vi "主界面B010 - 副本.vi"() -> ()   [LabVIEW 2013]
uses:
  <vilib>/Utility/file.llb/Read From Spreadsheet File (string).vi
  PCI8622_32.dll
panel:
  in  "Y挡圈最大值":dbl
  in  "Y挡圈最小值":dbl
  in  "X挡圈最大值":dbl
  in  "X挡圈最小值":dbl
  in  "Y内圈最大值":dbl
  in  "Y内圈最小值":dbl
  in  "X内圈最大值":dbl
  in  "X内圈最小值":dbl
  in  "Y轴承最大值":dbl
  in  "Y轴承最小值":dbl format="%#_13g"
  in  "X轴承最大值":dbl=12.0 format="%#_13g"
  in  "X轴承最小值":dbl=1.0 format="%#_13g"
  out "数值":i32
  out "员工ID":string
  out "压铆最大压力(N)":dbl
  out "压铆最小压力(N)":dbl
  out "3最大压装位移":dbl
  out "3最小压装位移":dbl
  out "3监控点":dbl
  in  "压轴承换向压力":dbl=5000.0
  out "换向指示1":bool
  in  "报警工步号":dbl
  out "报警提示":string
  in  "轴承压头速度（手动）":dbl
  in  "轴承压头位置（手动）":dbl
  in  "轴承内圈压头速度（手动）":dbl
  in  "轴承内圈压头位置（手动）":dbl
  out "换向指示2":bool
  in  "换向压力2":dbl=5000.0
  in  "工步号复位":bool
  out "通讯状态":bool
  in  "电动缸2ARST":bool
  in  "电动缸1ARST":bool
  out "内圈压头位置(mm)":dbl format="%#.1f"
  out "轴承压头位置(mm)":dbl format="%#.1f"
  out "型号数量":i32
  out "轴承压头位移(mm)":dbl format="%#.1f"
  out "内圈位移(mm)":dbl format="%#.1f"
  out "压铆位移(mm)":dbl format="%#.1f"
  out "压铆压力(N)":dbl format="%#.1f"
  out "error out 4":errorcluster
  out "error out 3":errorcluster
  out "error out 2":errorcluster
  out "ADODB._Connection Out":refnum<k7>
  out "error out":errorcluster
  out "B010本序不合格":bool
  out "内圈压力(N)":dbl format="%#.1f"
  out "轴承压头压力(N)":dbl format="%#.1f"
  out "B010本序合格":bool
  in  "停止":bool
  in  "自动工步号":dbl
  out "产品选型":dbl
  out "芯片ID":string
  out "自动操作状态":string
  in  "联线按钮":bool
  in  "选项卡控件":T1(tab)
  out "轴承区域最小压力(N)":dbl
  out "轴承区域最大压力(N)":dbl
  out "压轴承最大压力(N)":dbl
  out "轴承压装位移(mm)":dbl
  out "轴承最小压装位移(mm)":dbl
  out "轴承最大压装位移(mm)":dbl
  out "轴承监控点":dbl
  out "压装轴承，挡圈曲线":cluster{"Y":dbl[], "Y":dbl[]}[](graph) caption="压球涨堵头1"
  out "轴承最小压力(N)":dbl
  out "轴承最大压力(N)":dbl
  out "压装轴承合格":bool
  out "压装轴承不合格":bool
  out "轴承监控点压力(N)":dbl
  out "内圈区域压力最大值(N)":dbl
  out "内圈区域压力最小值(N)":dbl
  out "内圈压装最大压力(N)":dbl
  out "压装滚针轴承":cluster{"Y":dbl[], "Y":dbl[]}[](graph) caption="压球涨堵头1"
  out "压内圈不合格":bool
  out "压内圈合格":bool
  out "内圈最大压力(N)":dbl
  out "内圈最小压力(N)":dbl
  out "内圈监控点":dbl
  out "内圈最大压装位移(mm)":dbl
  out "内圈最小压装位移(mm)":dbl
  out "内圈实测压装位移(mm)":dbl
  out "内圈监控点压力(N)":dbl
  out "压铆区域内最大压力(N)":dbl
  out "压铆区域内最小压力(N)":dbl
  out "挡圈压铆":cluster{"Y":dbl[], "Y":dbl[]}[](graph) caption="压球涨堵头1"
  out "压挡圈合格":bool
  out "压挡圈不合格":bool
  out "压铆最大压力(N)":dbl
  out "压铆压装位移(mm)":dbl
  out "轴承正面":bool
  in  "伺服2P 启动":bool
  in  "伺服1P 启动":bool
  in  "快速上升速度":dbl
  in  "快速上升位置":dbl
  in  "慢速下降速度":dbl
  in  "慢速下降位置":dbl
  in  "快速下降速度":dbl
  in  "快速下降位置":dbl
  in  "快速上升速度":dbl
  in  "快速上升位置":dbl
  in  "慢速下降速度":dbl
  in  "慢速下降位置":dbl
  in  "快速下降速度":dbl
  in  "伺服2回零":bool
  in  "伺服2上升":bool
  in  "伺服2下降":bool
  in  "伺服2复位":bool
  in  "快速下降位置":dbl
  in  "伺服1回零":bool
  in  "伺服1上升":bool
  in  "伺服1下降":bool
  in  "伺服1复位":bool
  out "急停按钮":bool
  out "联线状态":bool
  out "光幕保护":bool
  out "气压报警":bool
  out "滑台右位":bool
  out "滑台左位":bool
  in  "滑台右移":bool
  in  "滑台左移":bool
  in  "增压缸下压":bool
  in  "增压缸上升":bool
  in  "增压缸增压":bool
  in  "增压缸卸压":bool
  in  "压铆压力零点偏移":dbl format="%#.2f"
  in  "压铆压力比例偏移":dbl format="%#.2f"
  in  "压铆位移零点偏移":dbl format="%#.2f"
  in  "压铆位移比例偏移":dbl format="%#.2f"
  in  "内圈压力零点偏移":dbl format="%#.2f"
  in  "内圈压力比例偏移":dbl format="%#.2f"
  in  "内圈位移零点偏移":dbl format="%#.2f"
  in  "内圈位移比例偏移":dbl format="%#.2f"
  in  "轴承压力零点偏移":dbl format="%#.2f"
  in  "轴承压力比例偏移":dbl format="%#.2f"
  in  "轴承位移零点偏移":dbl format="%#.2f"
  in  "轴承位移比例偏移":dbl format="%#.2f"
  in  "传感器参数查询":bool
  in  "传感器参数保存":bool
  in  "参数浏览表":string[][](table)=[["J709", "J728", "J706"], ["1", "1", "1"], ["168", "78.5", "98"], ["0", "500", "500"], ["10000", "5000", "5000"], ["0", "78", "97"], ["173", "80", "102"], ["183", "85.5", "79"], ["0", "500", "500"], ["20000", "5000", "5000"], ["0", "85.5", "83"], ["190", "86.5", "84"], ["250", "144", "144"], ["0", "55000", "55000"], ["100000", "65000", "65000"], ["0", "143", "143"], ["300", "147", "147"], ["-70", "-89\n", "-94"], ["20", "50", "50"], ["-80.95", "-104", "-113"], ["1", "1", "1"], ["0", "0", "0"], ["20", "50", "50"], ["-77", "-70", "-75"], ["20", "50", "50"], ["-92.5", "-82", "-87"], ["1", "1", "1"], ["0", "0", "0"], ["20", "50", "50"], ["1", "95", "97"], ["84", "96", "99"], ["2000", "500", "500"], ["4000", "5000", "5000"], ["81", "75", "79"], ["82", "77", "81"], ["0", "500", "500"], ["25000", "5000", "5000"], ["250", "184", "143"], ["252", "186", "144"], ["10000", "10000", "10000"], ["60000", "50000", "50000"], ["", "5000", "5000"], ["", "5000", "5000"], ["", "93", "93"], ["", "100", "102"], ["", "-10", "-10"], ["", "10000", "10000"], ["", "71", "77"], ["", "80", "85"], ["", "-10", "-10"], ["", "6000", "6000"], ["", "180", ""], ["", "190", ""], ["", "-10", ""], ["", "70000", ""]]
  in  "参数查询":bool
  in  "试验参数保存":bool
  in  "轴承区域最小位移(mm)":dbl=84.0
  in  "轴承区域最大位移(mm)":dbl=85.0
  in  "轴承区域最小压力(N)":dbl=500.0
  in  "轴承区域最大压力(N)":dbl=5000.0
  in  "内圈区域最小位移(mm)":dbl=90.0
  in  "内圈区域最大位移(mm)":dbl=91.0
  in  "内圈区域最小压力(N)":dbl=500.0
  in  "内圈区域最大压力(N)":dbl=5000.0
  in  "挡圈区域最小位移(mm)":dbl=250.0
  in  "挡圈区域最大位移(mm)":dbl=252.0
  in  "挡圈区域最小压力(N)":dbl=10000.0
  in  "挡圈区域最大压力(N)":dbl=60000.0
  out "员工姓名":string
  in  "型号选择":u16(ring)=1 items=["J709", "J728", "J706"]
  in  "参数加载":bool
  out "产品ID":string
  # "判定参数"
  # "芜湖机械转向器装配线"
  # "齿轮轴总成装配"
  # "Q14070机械转向器装配线"
  # "湖北唯思凌科装备制造有限公司 设计开发 (C)2015"
  # "判定参数"
  # "实测值"
  # "判定参数"
  # "实测值"
  # "实测值"
  # "轴承\n压头\n设置"
  # "轴承\n内圈\n压头\n设置"
  # "传感器校验区"
  # "注意：\n具备权限的用户才能够修改传感器校验参数和试验参数！"
  # "关于传感器校验：\n1、传感器校验需要由具备资质的单位或部门进行校验。\n2、具备权限的用户才能够修改传感器校验参数和试验参数。\n3、修改校验参数方法：先将比例偏移置为1，修改零点偏移，使零点值与校验的传感器一致；然后根据增幅调整比例偏移。"
  # "注意：\n具备权限的用户才能够修改传感器校验参数和试验参数！"
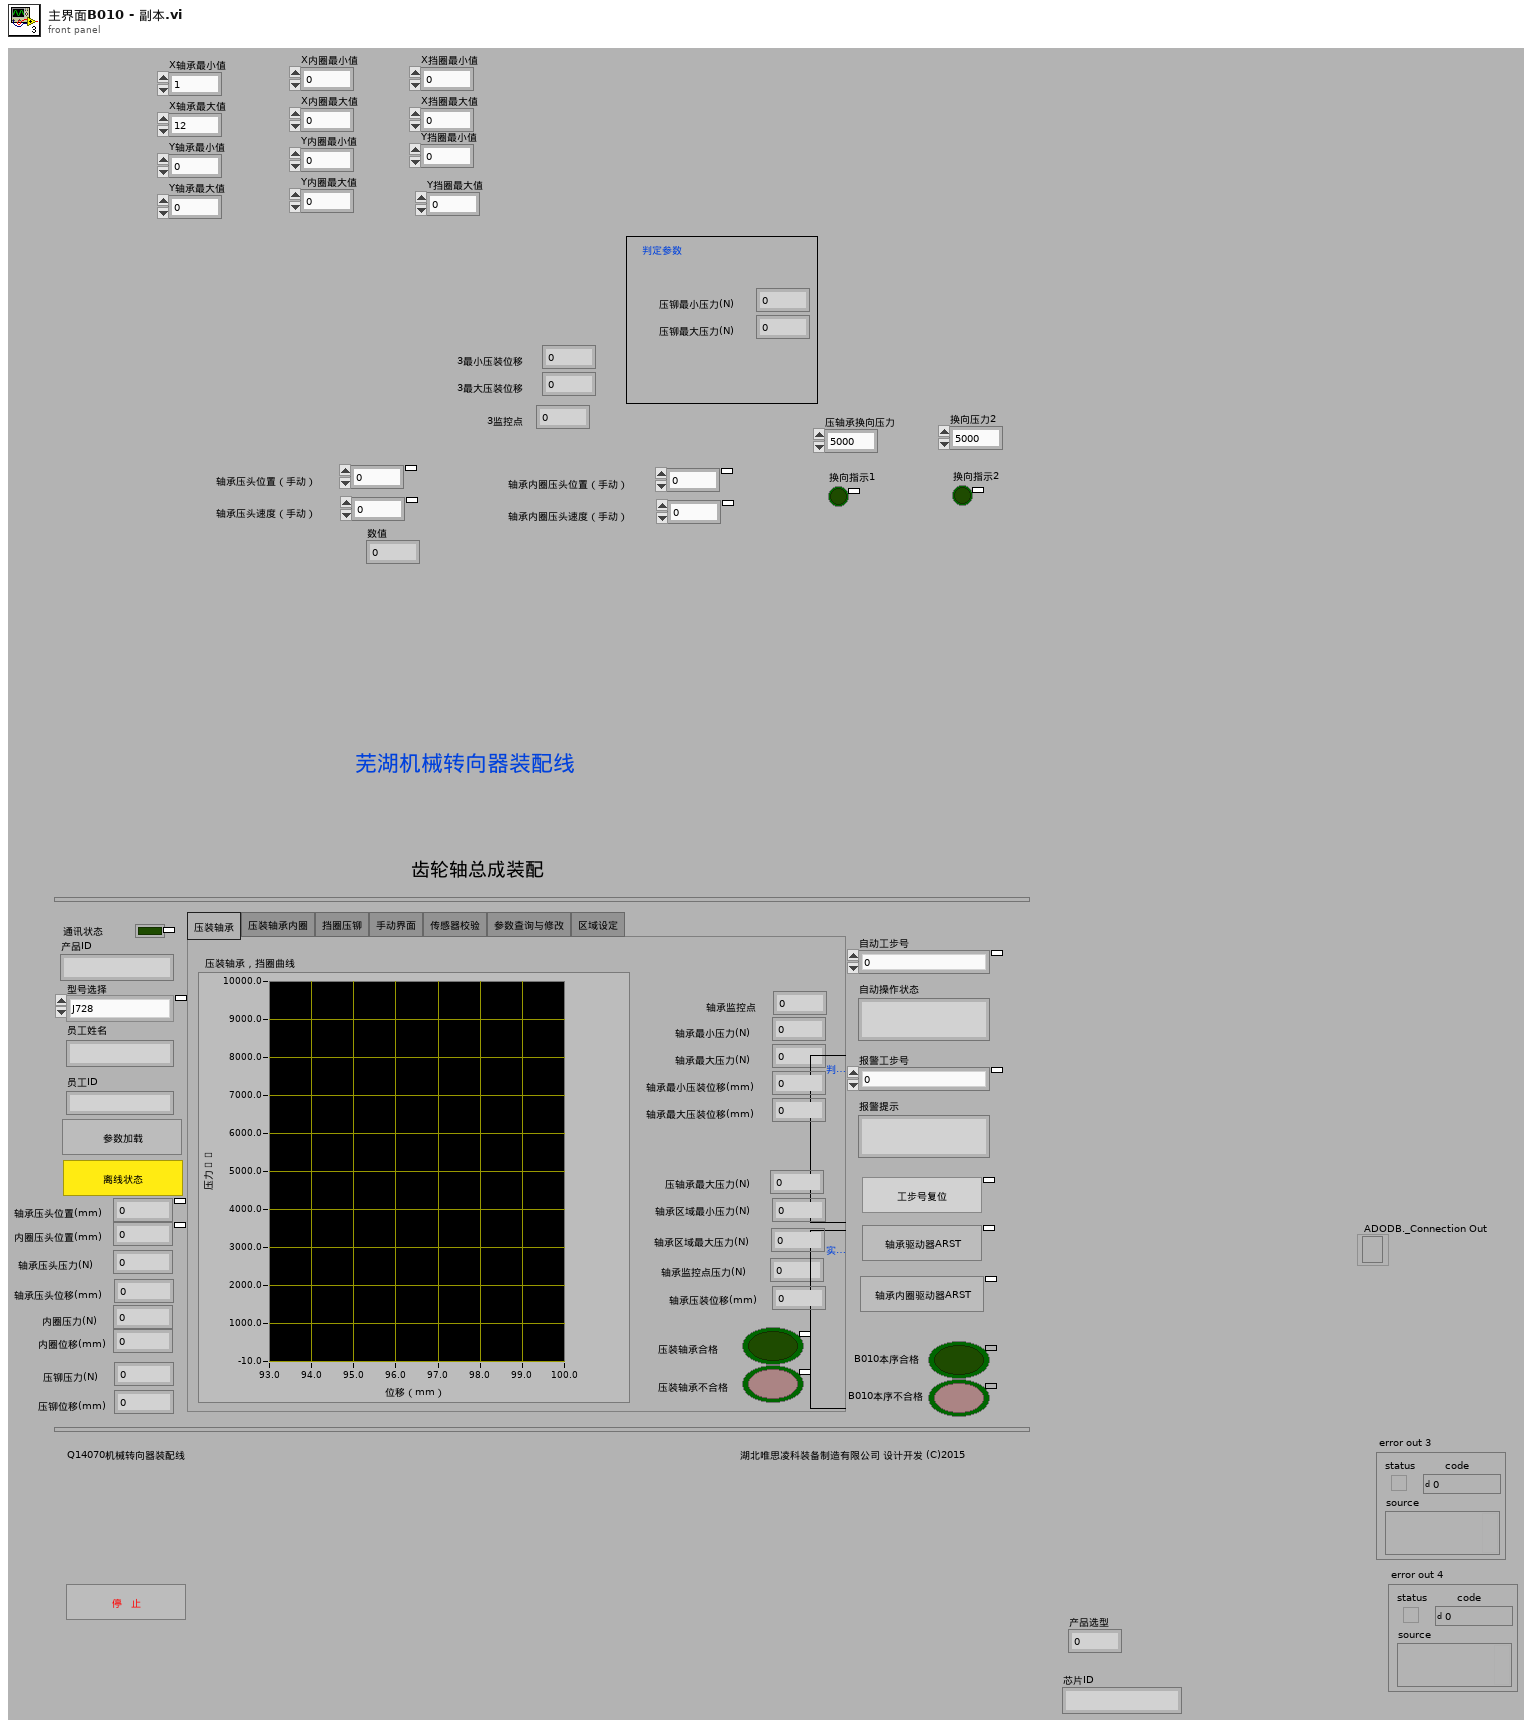
[diagram p1: front panel]
types:
  T1 = enum32{"压装轴承", "压装轴承内圈", "挡圈压铆", "手动界面", "传感器校验", "参数查询与修改", "区域设定"}
  T2 = typedef "imagedata.ctl" = cluster{"image type":i32, "image depth":i32, "image":u8[], "mask":u8[], "colors":u32[], "Rectangle":cluster{"left":i16, "top":i16, "right":i16, "bottom":i16}}
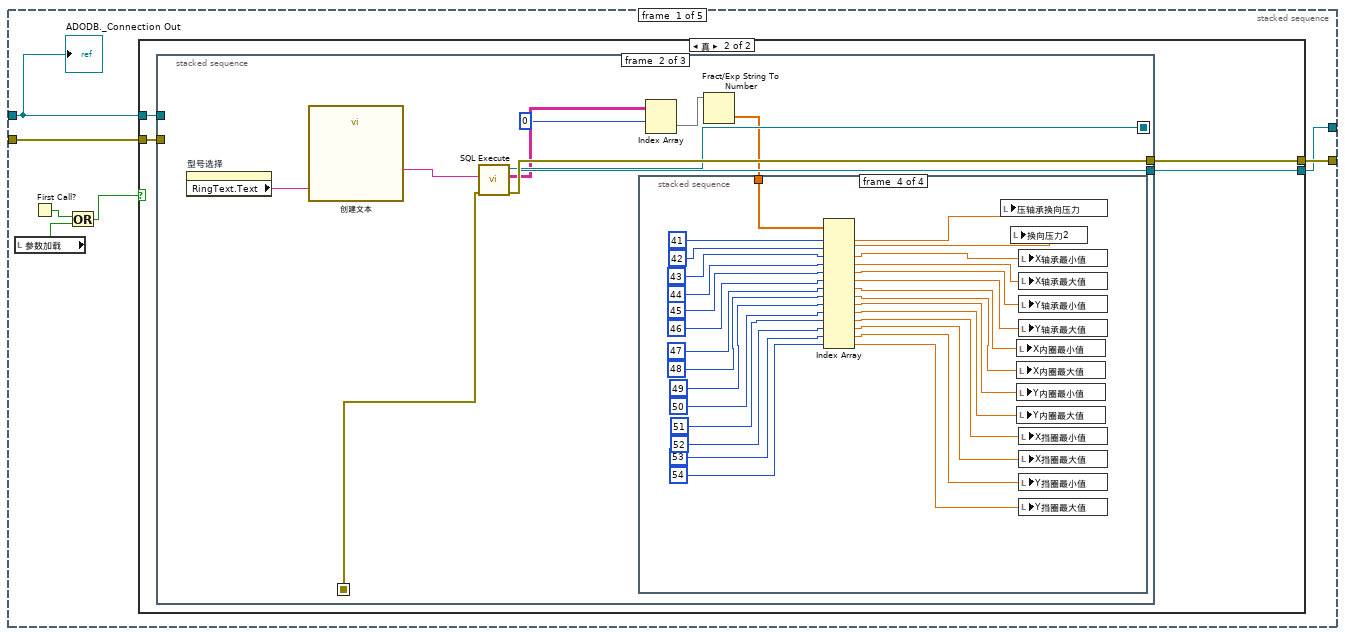
[diagram p2: hidden frame]
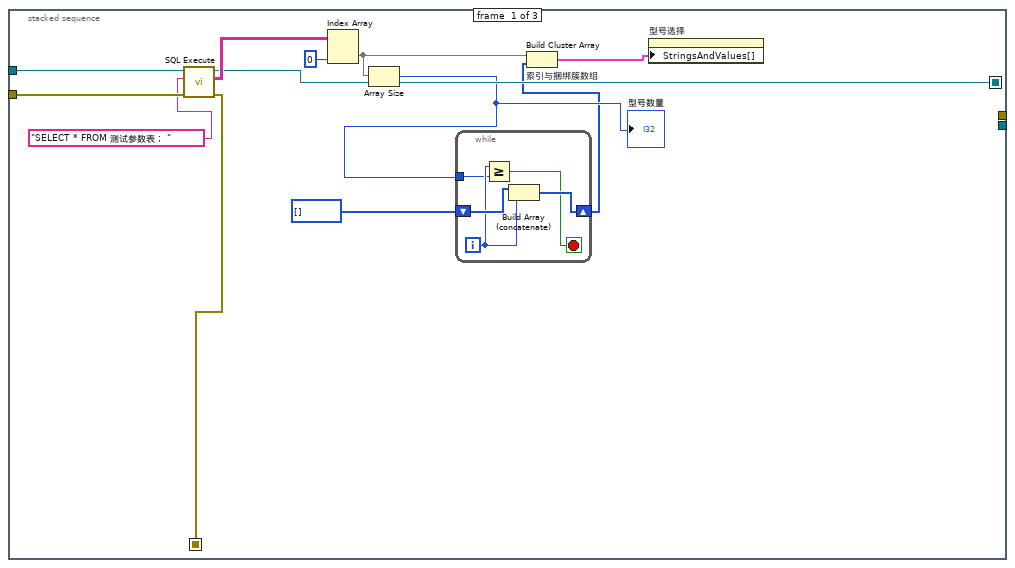
[diagram p4: hidden frame]
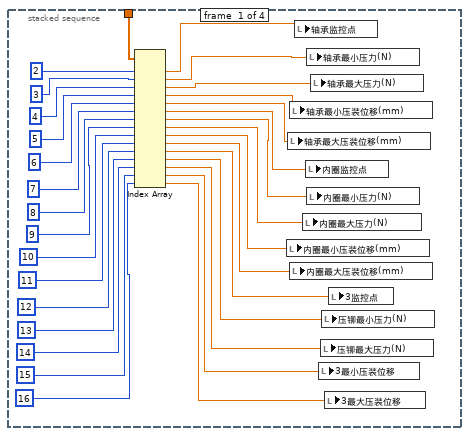
[diagram p5: hidden frame]
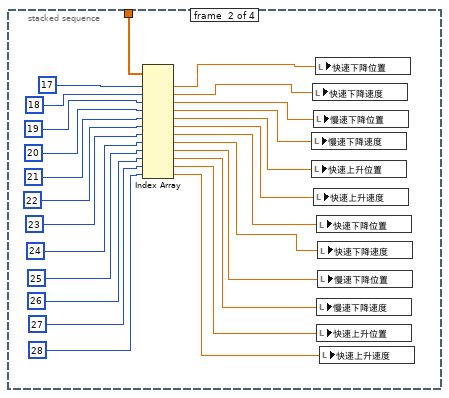
[diagram p6: hidden frame]
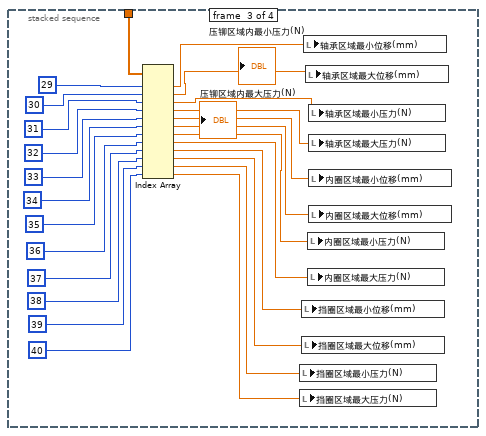
[diagram p7: hidden frame]
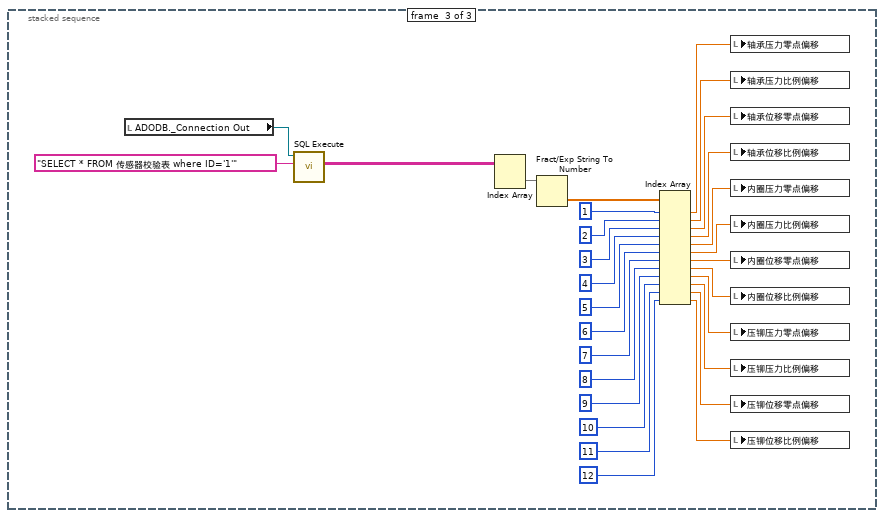
[diagram p8: hidden frame]
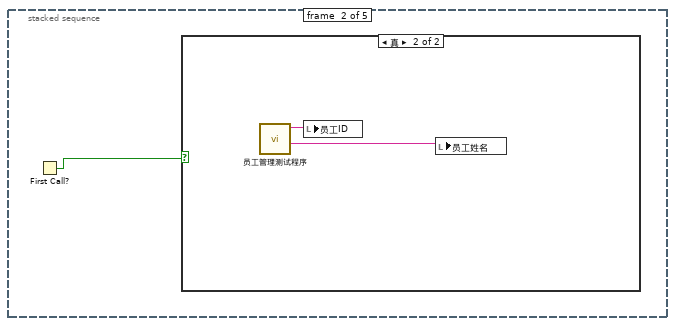
[diagram p9: hidden frame]
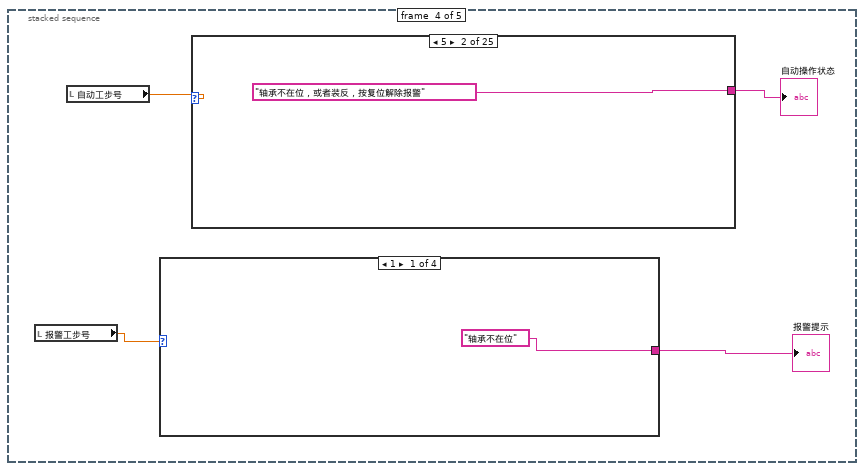
[diagram p11: hidden frame]
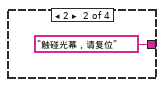
[diagram p12: hidden frame]
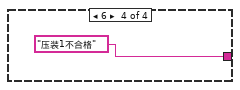
[diagram p14: hidden frame]
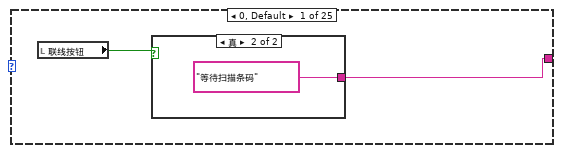
[diagram p15: hidden frame]
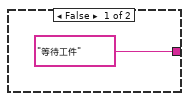
[diagram p16: hidden frame]
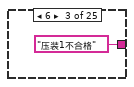
[diagram p17: hidden frame]
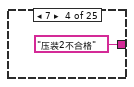
[diagram p18: hidden frame]
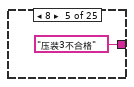
[diagram p19: hidden frame]
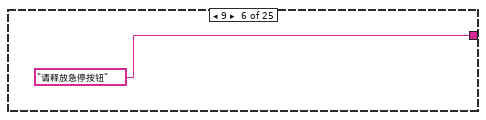
[diagram p20: hidden frame]
diagram:
  n1 = while {
    stop <- w10 stop-if-true
    n2 = local read "自动工步号"() -> (w8:dbl)
    n3 = Wait Until Next ms Multiple(millisecond multiple=u32 100 ("毫秒倍数")) -> ()  [unwired: 1 out]
    n4 = case shown="60" w8 {
      frame 0, Default {
      }
      frame 10 {
        n5 = flat-sequence {
          tunnel: [w25] -> w16
          tunnel: [w33] -> w22
          tunnel: [w32] -> w21
          tunnel: w16 -> [w31]
          tunnel: w22 -> [w59]
          tunnel: w21 -> [w57]
          tunnel: [w65] -> w20
          tunnel: [w64] -> w19
          tunnel: [w58] -> w14
          tunnel: w20 -> [w73]
          tunnel: w19 -> [w78]
          tunnel: [w75] -> w18
          tunnel: [w71] -> w17
          tunnel: [w70] -> w15
          tunnel: w14 -> [w70]
          tunnel: [w69] -> w13
          tunnel: [w68] -> w12
          tunnel: w18 -> [w87]
          tunnel: w17 -> [w86]
          tunnel: w15 -> [w83]
          tunnel: w13 -> [w85]
          tunnel: w12 -> [w84]
          tunnel: [w79] -> w11
          tunnel: w11 -> [w89]
          frame #0 {
            w23 = FALSE ("换向指示1")
            w30 = FALSE
            n6 = local write "压装轴承不合格"(w30) -> ()
            n7 = local write "压装轴承合格"(w30) -> ()
            n8 = property on="轴承监控点压力(N)" class="DigNum (严格)"("Blinking"=w23) -> ()  [unwired: 2 in, 2 out]
            n9 = local write "换向指示1"(w23) -> ()
            n10 = local write "换向指示2"(w23) -> ()
            n11 = local write "选项卡控件"(T1."压装轴承" ("选项卡控件")) -> ()
            n12 = call "区域曲线.vi"("区域最大压力(N)"="轴承区域最大压力(N)", "区域最小压力(N)"="轴承区域最小压力(N)", "区域最大位移(mm)"="轴承区域最大位移(mm)", "区域最小位移(mm)"="轴承区域最小位移(mm)") -> ("区域曲线"=w25:cluster{dbl[], dbl[]})  [unwired: 7 in]
          }
          frame #1 {
            w34 = dbl[] []
            n13 = while {
              shift-right: [w52] -> w33
              shift-left: w34 -> [w53]
              shift-right: [w50] -> w32
              shift-left: w34 -> [w51]
              tunnel: w31 -> [w40]
              stop <- w36 stop-if-true
              n14 = local read "轴承压头位置(mm)"() -> (w43:dbl)
              n15 = local read "自动工步号"() -> (w46:dbl)
              n16 = local read "轴承压头压力(N)"() -> (w49:dbl)
              n17 = local read "轴承压头压力(N)"() -> (w39:dbl)
              n18 = local read "压轴承换向压力"() -> (w38:dbl)
              n19 = Equal?(x=w46, y=30.0) -> (x = y?=w37:bool)
              n20 = Multiply(x=w43, y=-1.0) -> (x*y=w41:dbl)
              n21 = Build Array (concatenate)(w53, w41) -> (w52:dbl[])
              n22 = Build Array (concatenate)(w51, w49) -> (w50:dbl[])
              n23 = Bundle(w52, w50) -> (w48:cluster{dbl[], dbl[]})  [unwired: 1 in]
              n24 = Greater Or Equal?(x=w39, y=w38) -> (x >= y?=w35:bool)
              n25 = Build Array(w48, w40) -> (w47:cluster{dbl[], dbl[]}[])
              n26 = Or(x=w37, y=w35) -> (x .or. y?=w36:bool)
              n27 = local write "压装轴承，挡圈曲线"(w47) -> ()
              n28 = Wait Until Next ms Multiple(millisecond multiple=u32 50 ("毫秒倍数")) -> ()  [unwired: 1 out]
              n29 = local write "换向指示1"(w35) -> ()
            }
          }
          frame #2 {
            n30 = local read "轴承监控点"() -> (w67:dbl)
            n31 = local read "轴承区域最大位移(mm)"() -> (w62:dbl)
            n32 = local read "轴承区域最小位移(mm)"() -> (w63:dbl)
            n33 = local read "轴承区域最小压力(N)"() -> (w61:dbl)
            n34 = local read "轴承区域最大压力(N)"() -> (w60:dbl)
            n35 = Array Max & Min(array=w59) -> (max value=w64:dbl)  [unwired: 3 out]
            n36 = Array Max & Min(array=w57) -> (max value=→"压轴承最大压力(N)":dbl)  [unwired: 3 out]
            n37 = Threshold 1D Array "以阈值插值一维数组"(2:w67, 3:w59) -> (0:w66:dbl)  [unwired: 1 in]
            n38 = local write "轴承压装位移(mm)"(w64) -> ()
            n39 = Index Array(array=w57, index=w66) -> (element=w65:dbl)
            n40 = call "区域判断.vi"("压力数组"=w57, "位移数组"=w59, "区域最大压力"=w60, "区域最小压力"=w61, "区域最大位移"=w62, "区域最小位移"=w63) -> ("数值 2"=→"轴承区域最小压力(N)":dbl, "数值"=→"轴承区域最大压力(N)":dbl, "区域监控合格"=w58:bool)  [unwired: 1 in]
            n41 = local write "轴承监控点压力(N)"(w65) -> ()
          }
          frame #3 {
            n42 = local read "轴承最大压装位移(mm)"() -> (w77:dbl)
            n43 = local read "轴承最小压装位移(mm)"() -> (w76:dbl)
            n44 = local read "轴承最大压力(N)"() -> (w72:dbl)
            n45 = local read "轴承最小压力(N)"() -> (w74:dbl)
            n46 = In Range and Coerce(upper limit=w77, x=w78, lower limit=w76) -> (In Range?=w69:bool)  [unwired: 1 out]
            n47 = In Range and Coerce(upper limit=w72, x=w73, lower limit=w74) -> (In Range?=w68:bool)  [unwired: 1 out]
            n48 = Not(x=w69) -> (.not. x?=w75:bool)
            n49 = Not(x=w68) -> (.not. x?=w71:bool)
          }
          frame #4 {
            n50 = property on="轴承监控点压力(N)" class="DigNum (严格)"("Blinking"=w86) -> ()  [unwired: 2 in, 2 out]
            n51 = property on="轴承压装位移(mm)" class="DigNum (严格)"("Blinking"=w87) -> ()  [unwired: 2 in, 2 out]
            n52 = Compound Arithmetic op=AND(w85, w84, w83) -> (w82:bool)
            "压装轴承合格" <- w82
            n53 = Not(x=w82) -> (.not. x?=w81:bool)
            "压装轴承不合格" <- w81
            n54 = Wait Until Next ms Multiple(millisecond multiple=u32 80 ("毫秒倍数")) -> ()  [unwired: 1 out]
            n55 = local read "联线按钮"() -> (w80:bool)
            n56 = And(x=w81, y=w80) -> (x .and. y?=w79:bool)
          }
          frame #5 {
            n57 = case shown="真" w89 {
              frame False {
              }
              frame True {
                n58 = local write "B010本序不合格"(TRUE ("B010本序不合格")) -> ()
                n59 = local write "B010本序合格"(FALSE ("B010本序合格")) -> ()
              }
            }
          }
        }
      }
      frame 60 {
        n60 = flat-sequence {
          tunnel: [w107] -> w98
          tunnel: [w114] -> w104
          tunnel: [w113] -> w103
          tunnel: w98 -> [w112]
          tunnel: w104 -> [w140]
          tunnel: w103 -> [w138]
          tunnel: [w146] -> w102
          tunnel: [w145] -> w101
          tunnel: [w139] -> w96
          tunnel: w102 -> [w157]
          tunnel: w101 -> [w159]
          tunnel: [w158] -> w100
          tunnel: [w156] -> w99
          tunnel: [w151] -> w97
          tunnel: w96 -> [w151]
          tunnel: [w150] -> w95
          tunnel: [w149] -> w94
          tunnel: w100 -> [w167]
          tunnel: w99 -> [w166]
          tunnel: w97 -> [w165]
          tunnel: w95 -> [w164]
          tunnel: w94 -> [w163]
          tunnel: [w161] -> w93
          tunnel: [w160] -> w92
          tunnel: w93 -> [w171]
          tunnel: w92 -> [w170]
          frame #0 {
            w105 = FALSE
            n61 = property on="内圈监控点压力(N)" class="DigNum (严格)"("Blinking"=w105) -> ()  [unwired: 2 in, 2 out]
            n62 = local write "压内圈合格"(w105) -> ()
            n63 = local write "压内圈不合格"(w105) -> ()
            n64 = local write "换向指示2"(w105) -> ()
            n65 = local write "选项卡控件"(T1."压装轴承内圈" ("选项卡控件")) -> ()
            n66 = call "区域曲线.vi"("区域最大压力(N)"="内圈区域最大压力(N)", "区域最小压力(N)"="内圈区域最小压力(N)", "区域最大位移(mm)"="内圈区域最大位移(mm)", "区域最小位移(mm)"="内圈区域最小位移(mm)") -> ("区域曲线"=w107:cluster{dbl[], dbl[]})  [unwired: 7 in]
          }
          frame #1 {
            w115 = dbl[] []
            n67 = while {
              shift-right: [w133] -> w114
              shift-left: w115 -> [w134]
              shift-right: [w131] -> w113
              shift-left: w115 -> [w132]
              tunnel: w112 -> [w120]
              stop <- w119 stop-if-true
              n68 = local read "内圈压头位置(mm)"() -> (w122:dbl)
              n69 = local read "内圈压力(N)"() -> (w118:dbl)
              n70 = local read "内圈压力(N)"() -> (w121:dbl)
              n71 = local read "自动工步号"() -> (w129:dbl)
              n72 = Multiply(x=w122, y=-1.0) -> (x*y=w125:dbl)
              n73 = Build Array (concatenate)(w134, w125) -> (w133:dbl[])
              n74 = Build Array (concatenate)(w132, w121) -> (w131:dbl[])
              n75 = Equal?(x=w129, y=80.0) -> (x = y?=w127:bool)
              n76 = Greater Or Equal?(x=w118, y="换向压力2") -> (x >= y?=w116:bool)
              n77 = Or(x=w116, y=w127) -> (x .or. y?=w119:bool)
              n78 = Bundle(w133, w131) -> (w130:cluster{dbl[], dbl[]})  [unwired: 1 in]
              n79 = local write "换向指示2"(w116) -> ()
              n80 = Build Array(w130, w120) -> (w124:cluster{dbl[], dbl[]}[])
              n81 = local write "压装滚针轴承"(w124) -> ()
              n82 = Wait Until Next ms Multiple(millisecond multiple=u32 50 ("毫秒倍数")) -> ()  [unwired: 1 out]
            }
          }
          frame #2 {
            n83 = local read "内圈监控点"() -> (w147:dbl)
            n84 = local read "内圈区域最小位移(mm)"() -> (w144:dbl)
            n85 = local read "内圈区域最大位移(mm)"() -> (w143:dbl)
            n86 = local read "内圈区域最小压力(N)"() -> (w142:dbl)
            n87 = local read "内圈区域最大压力(N)"() -> (w141:dbl)
            n88 = Array Max & Min(array=w140) -> (max value=w145:dbl)  [unwired: 3 out]
            n89 = Array Max & Min(array=w138) -> (max value=→"内圈压装最大压力(N)":dbl)  [unwired: 3 out]
            n90 = Threshold 1D Array(2:w147, 3:w140) -> (0:w148:dbl)  [unwired: 1 in]
            n91 = Index Array(array=w138, index=w148) -> (element=w146:dbl)
            n92 = local write "内圈实测压装位移(mm)"(w145) -> ()
            n93 = local write "内圈监控点压力(N)"(w146) -> ()
            n94 = call "区域判断.vi"("压力数组"=w138, "位移数组"=w140, "区域最大压力"=w141, "区域最小压力"=w142, "区域最大位移"=w143, "区域最小位移"=w144) -> ("数值 2"=→"内圈区域压力最小值(N)":dbl, "数值"=→"内圈区域压力最大值(N)":dbl, "区域监控合格"=w139:bool)  [unwired: 1 in]
          }
          frame #3 {
            n95 = local read "内圈最大压装位移(mm)"() -> (w154:dbl)
            n96 = local read "内圈最小压装位移(mm)"() -> (w155:dbl)
            n97 = local read "内圈最大压力(N)"() -> (w153:dbl)
            n98 = local read "内圈最小压力(N)"() -> (w152:dbl)
            n99 = In Range and Coerce(upper limit=w154, x=w159, lower limit=w155) -> (In Range?=w150:bool)  [unwired: 1 out]
            n100 = In Range and Coerce(upper limit=w153, x=w157, lower limit=w152) -> (In Range?=w149:bool)  [unwired: 1 out]
            n101 = Not(x=w150) -> (.not. x?=w158:bool)
            n102 = Not(x=w149) -> (.not. x?=w156:bool)
          }
          frame #4 {
            n103 = property on="内圈监控点压力(N)" class="DigNum (严格)"("Blinking"=w166) -> ()  [unwired: 2 in, 2 out]
            n104 = property on="内圈实测压装位移(mm)" class="DigNum (严格)"("Blinking"=w167) -> ()  [unwired: 2 in, 2 out]
            n105 = Compound Arithmetic op=AND(w164, w165, w163) -> (w162:bool)
            n106 = Not(x=w162) -> (.not. x?=w161:bool)
            n107 = Wait Until Next ms Multiple(millisecond multiple=u32 80 ("毫秒倍数")) -> ()  [unwired: 1 out]
            n108 = local write "压内圈合格"(w162) -> ()
            n109 = local write "压内圈不合格"(w161) -> ()
            n110 = local read "联线按钮"() -> (w160:bool)
          }
          frame #5 {
            n111 = And(x=w171, y=w170) -> (x .and. y?=w169:bool)
            n112 = case shown="真" w169 {
              frame False {
              }
              frame True {
                n113 = local write "B010本序不合格"(TRUE ("B010本序不合格")) -> ()
                n114 = local write "B010本序合格"(FALSE ("B010本序合格")) -> ()
              }
            }
          }
        }
      }
      frame 110 {
        n115 = flat-sequence {
          tunnel: [w202] -> w190
          tunnel: [w194] -> w175
          tunnel: [w207] -> w193
          tunnel: [w206] -> w192
          tunnel: w190 -> [w205]
          tunnel: w175 -> [w204]
          tunnel: w193 -> [w227]
          tunnel: w192 -> [w228]
          tunnel: [w235] -> w183
          tunnel: [w236] -> w181
          tunnel: [w232] -> w179
          tunnel: [w231] -> w177
          tunnel: w183 -> [w242]
          tunnel: [w242] -> w182
          tunnel: w181 -> [w241]
          tunnel: [w241] -> w180
          tunnel: w179 -> [w240]
          tunnel: [w240] -> w178
          tunnel: w177 -> [w239]
          tunnel: [w239] -> w176
          tunnel: w182 -> [w255]
          tunnel: w180 -> [w257]
          tunnel: [w256] -> w191
          tunnel: w178 -> [w250]
          tunnel: [w250] -> w189
          tunnel: [w249] -> w188
          tunnel: [w248] -> w187
          tunnel: w176 -> [w245]
          tunnel: [w244] -> w184
          tunnel: [w243] -> w174
          tunnel: w191 -> [w266]
          tunnel: w189 -> [w260]
          tunnel: w188 -> [w261]
          tunnel: w187 -> [w265]
          tunnel: [w263] -> w186
          tunnel: [w262] -> w185
          tunnel: w184 -> [w259]
          tunnel: w174 -> [w258]
          tunnel: w186 -> [w270]
          tunnel: w185 -> [w269]
          frame #0 {
            w203 = FALSE
            n116 = local write "压挡圈不合格"(w203) -> ()
            n117 = local write "压挡圈合格"(w203) -> ()
            n118 = local write "选项卡控件"(T1."挡圈压铆" ("选项卡控件")) -> ()
            n119 = call "区域曲线.vi"("区域最大压力(N)"="挡圈区域最大压力(N)", "区域最小压力(N)"="挡圈区域最小压力(N)", "区域最大位移(mm)"="挡圈区域最大位移(mm)", "区域最小位移(mm)"="挡圈区域最小位移(mm)") -> ("区域曲线"=w202:cluster{dbl[], dbl[]})  [unwired: 7 in]
            n120 = call "区域曲线 - 副本.vi"("区域最大压力(N)"=100000.0, "区域最小压力(N)"=0.0, "区域最大位移(mm)"="挡圈区域最大位移(mm)", "区域最小位移(mm)"="挡圈区域最小位移(mm)") -> ("区域曲线1"=w194:cluster{dbl[], dbl[]})  [unwired: 7 in]
          }
          frame #1 {
            w208 = dbl[] []
            n121 = while {
              shift-right: [w211] -> w207
              shift-left: w208 -> [w223]
              shift-right: [w210] -> w206
              shift-left: w208 -> [w222]
              tunnel: w205 -> [w213]
              tunnel: w204 -> [w209]
              stop <- w218 stop-if-true
              n122 = local read "压铆压力(N)"() -> (w215:dbl)
              n123 = local read "压铆位移(mm)"() -> (w216:dbl)
              n124 = local read "自动工步号"() -> (w220:dbl)
              n125 = Build Array (concatenate)(w223, w216) -> (w211:dbl[])
              n126 = Build Array (concatenate)(w222, w215) -> (w210:dbl[])
              n127 = Equal?(x=w220, y=140.0) -> (x = y?=w218:bool)
              n128 = Bundle(w211, w210) -> (w221:cluster{dbl[], dbl[]})  [unwired: 1 in]
              n129 = Build Array(w221) -> (w214:cluster{dbl[], dbl[]}[])
              n130 = Build Array (concatenate)(w214, w213, w209) -> (w212:cluster{dbl[], dbl[]}[])
              n131 = Wait Until Next ms Multiple(millisecond multiple=u32 2 ("毫秒倍数")) -> ()  [unwired: 1 out]
              n132 = local write "挡圈压铆"(w212) -> ()
            }
          }
          frame #2 {
            n133 = local read "挡圈区域最小位移(mm)"() -> (w230:dbl)
            n134 = local read "挡圈区域最大位移(mm)"() -> (w229:dbl)
            n135 = local read "挡圈区域最大压力(N)"() -> (w233:dbl)
            n136 = local read "挡圈区域最小压力(N)"() -> (w234:dbl)
            n137 = local read "3监控点"() -> (w237:dbl)
            n138 = Array Max & Min(array=w227) -> (max value=w236:dbl)  [unwired: 3 out]
            n139 = Threshold 1D Array(2:w237, 3:w227) -> (0:w238:dbl)  [unwired: 1 in]
            n140 = Index Array(array=w228, index=w238) -> (element=w235:dbl)
            n141 = call "区域判断.vi"("压力数组"=w228, "位移数组"=w227, "区域最大压力"=w233, "区域最小压力"=w234, "区域最大位移"=w229, "区域最小位移"=w230) -> ("数值 2"=w226:dbl, "数值"=w225:dbl, "区域监控合格"=w232:bool)  [unwired: 1 in]
            n142 = local write "压铆压装位移(mm)"(w236) -> ()
            n143 = local write "压铆区域内最小压力(N)"(w226) -> ()
            n144 = local write "压铆区域内最大压力(N)"(w225) -> ()
            n145 = Array Max & Min(array=w228) -> (max value=w231:dbl)  [unwired: 3 out]
            n146 = local write "压铆最大压力(N)"(w231) -> ()
            n147 = property on="压铆最大压力(N)" class="DigNum (严格)"("Blinking"=FALSE ("闪烁")) -> ()  [unwired: 2 in, 2 out]
          }
          frame #3 {
          }
          frame #4 {
            n148 = local read "压铆最小压力(N)"() -> (w246:dbl)
            n149 = local read "挡圈区域最小压力(N)"() -> (w251:dbl)
            n150 = local read "压铆最大压力(N)"() -> (w247:dbl)
            n151 = local read "3最大压装位移"() -> (w254:dbl)
            n152 = local read "挡圈区域最大压力(N)"() -> (w252:dbl)
            n153 = local read "3最小压装位移"() -> (w253:dbl)
            n154 = In Range and Coerce(upper limit=w254, x=w257, lower limit=w253) -> (In Range?=w249:bool)  [unwired: 1 out]
            n155 = In Range and Coerce(upper limit=w252, x=w255, lower limit=w251) -> (In Range?=w248:bool)  [unwired: 1 out]
            n156 = In Range and Coerce(upper limit=w247, x=w245, lower limit=w246) -> (In Range?=w244:bool)  [unwired: 1 out]
            n157 = Not(x=w249) -> (.not. x?=w256:bool)
            n158 = Not(x=w244) -> (.not. x?=w243:bool)
          }
          frame #5 {
            n159 = property on="压铆最大压力(N)" class="DigNum (严格)"("Blinking"=w258) -> ()  [unwired: 2 in, 2 out]
            n160 = property on="压铆压装位移(mm)" class="DigNum (严格)"("Blinking"=w266) -> ()  [unwired: 2 in, 2 out]
            n161 = Compound Arithmetic op=AND(w265, w261, w260, w259) -> (w264:bool)
            n162 = Not(x=w264) -> (.not. x?=w263:bool)
            n163 = Wait Until Next ms Multiple(millisecond multiple=u32 80 ("毫秒倍数")) -> ()  [unwired: 1 out]
            n164 = local read "联线按钮"() -> (w262:bool)
            n165 = local write "压挡圈不合格"(w263) -> ()
            n166 = local write "压挡圈合格"(w264) -> ()
          }
          frame #6 {
            n167 = And(x=w270, y=w269) -> (x .and. y?=w268:bool)
            n168 = case shown="真" w268 {
              frame False {
              }
              frame True {
                n169 = local write "B010本序不合格"(TRUE ("B010本序不合格")) -> ()
                n170 = local write "B010本序合格"(FALSE ("B010本序合格")) -> ()
              }
            }
          }
        }
      }
      frame 150 {
        n171 = flat-sequence {
          tunnel: ["F:\\报表储存\\"] -> w289
          tunnel: [w297] -> w288
          tunnel: [w296] -> w287
          tunnel: [w295] -> w286
          tunnel: [w293] -> w285
          tunnel: w289 -> [w324]
          tunnel: w288 -> [w323]
          tunnel: w287 -> [w322]
          tunnel: w286 -> [w321]
          tunnel: w285 -> [w310]
          tunnel: [w319] -> w284
          tunnel: [w318] -> w283
          tunnel: [w313] -> w281
          tunnel: [w312] -> w277
          tunnel: w284 -> [w328]
          tunnel: w283 -> [w327]
          tunnel: [w327] -> w282
          tunnel: w281 -> [w326]
          tunnel: [w326] -> w280
          tunnel: w277 -> [w325]
          tunnel: [w325] -> w276
          tunnel: w282 -> [w333]
          tunnel: w280 -> [w332]
          tunnel: [w332] -> w279
          tunnel: w276 -> [w331]
          tunnel: [w331] -> w275
          tunnel: w279 -> [w337]
          tunnel: [w337] -> w278
          tunnel: w275 -> [w336]
          tunnel: [w336] -> w274
          tunnel: w278 -> [w341]
          tunnel: w274 -> [w339]
          tunnel: [w339] -> w273
          tunnel: w273 -> [w347]
          frame #0 {
            n172 = Wait (ms)(milliseconds to wait=u32 500 ("毫秒倍数")) -> ()  [unwired: 1 out]
          }
          frame #1 {
            n173 = local read "数值"() -> (w292:i32)
            n174 = Increment(x=w292) -> (x+1=→"数值":i32)
          }
          frame #2 {
            n175 = local read "数值"() -> (w294:i32)
            n176 = Format Date/Time String(time format string (%c)="%Y%m%d") -> (date/time string=w299:string)  [unwired: 2 in]
            n177 = String Subset(string=w299, offset (0)=6 ("偏移量(0)"), length (rest)=2 ("长度（剩余）")) -> (substring=w295:string)
            n178 = String Subset(string=w299, offset (0)=0 ("偏移量(0)"), length (rest)=4 ("长度（剩余）")) -> (substring=w297:string)
            n179 = String Subset(string=w299, offset (0)=4 ("偏移量(0)"), length (rest)=2 ("长度（剩余）")) -> (substring=w296:string)
            n180 = Number To Decimal String(number=w294) -> (decimal integer string=w293:string)  [unwired: 1 in]
          }
          frame #3 {
            w307 = "\\"
            n181 = Concatenate Strings(w324, w323, w307, w322, w307, w321, w307, w310, w307) -> (w320:string)
            n182 = Concatenate Strings(w324, w323, w307, w322, w307, w321, w307, w310, w307) -> (w311:string)
            n183 = String To Path(string=w320) -> (path=w319:path)
            n184 = Concatenate Strings(w311, w310, "轴承.JPG" ("字符串")) -> (w314:string)
            n185 = Concatenate Strings(w311, w310, "内圈.JPG" ("字符串")) -> (w315:string)
            n186 = Concatenate Strings(w311, w310, "挡圈.JPG" ("字符串")) -> (w317:string)
            n187 = String To Path(string=w314) -> (path=w312:path)
            n188 = String To Path(string=w315) -> (path=w313:path)
            n189 = String To Path(string=w317) -> (path=w318:path)
          }
          frame #4 {
            n190 = call <vilib>:"Check if File or Folder Exists.vi"("path"=w328) -> ("file or folder exists?"=w329:bool)  [unwired: 8 in, 2 out]
            n191 = case shown="假" w329 {
              tunnel: w328 -> [w330 _]
              frame False {
                n192 = Create Folder(path (use dialog)=w330) -> ()  [unwired: 2 in, 3 out]
              }
              frame True {
              }
            }
          }
          frame #5 {
            n193 = control-ref of="本VI"() -> (w335:refnum<vi>)
            n194 = invoke class="VI" method="FP.Get Image"(reference=w335) -> ("image data"=w334:T2)  [unwired: 5 in, 5 out]
            n195 = call <vilib>:"Write JPEG File.vi"("image data"=w334, "path to JPEG file"=w333) -> ()  [unwired: 8 in, 2 out]
          }
          frame #6 {
            n196 = Wait (ms)(milliseconds to wait=u32 500 ("毫秒倍数")) -> ()  [unwired: 1 out]
          }
          frame #7 {
            n197 = flat-sequence {
              tunnel: w341 -> [w342]
              tunnel: [w342] -> w340
              tunnel: w340 -> [w345]
              frame #0 {
                n198 = local write "选项卡控件"(T1."压装轴承内圈" ("选项卡控件")) -> ()
              }
              frame #1 {
                n199 = control-ref of="本VI"() -> (w346:refnum<vi>)
                n200 = invoke class="VI" method="FP.Get Image"(reference=w346) -> ("image data"=w344:T2)  [unwired: 5 in, 5 out]
                n201 = call <vilib>:"Write JPEG File.vi"("image data"=w344, "path to JPEG file"=w345) -> ()  [unwired: 8 in, 2 out]
              }
            }
          }
          frame #8 {
            n202 = flat-sequence {
              tunnel: w347 -> [w349]
              frame #0 {
                n203 = local write "选项卡控件"(T1."压装轴承" ("选项卡控件")) -> ()
              }
              frame #1 {
                n204 = control-ref of="本VI"() -> (w351:refnum<vi>)
                n205 = invoke class="VI" method="FP.Get Image"(reference=w351) -> ("image data"=w350:T2)  [unwired: 5 in, 5 out]
                n206 = call <vilib>:"Write JPEG File.vi"("image data"=w350, "path to JPEG file"=w349) -> ()  [unwired: 8 in, 2 out]
              }
            }
          }
          frame #9 {
            n207 = Wait (ms)(milliseconds to wait=u32 50 ("毫秒倍数")) -> ()  [unwired: 1 out]
            n208 = local write "选项卡控件"(T1."挡圈压铆" ("选项卡控件")) -> ()
          }
        }
      }
    }
    n209 = local read "停止"() -> (w10:bool)
  }
  n210 = while {
    stop <- w354 stop-if-true
    n211 = event shown="[1] \"参数加载\": 值改变" {
      selector: _ -> [_ _ _ _ _ _ _]
      dyn-events: _ -> [_ _ _ _ _ _ _]
      timeout: 500 -> [_ _ _ _ _ _ _]
      event Timeout {
        n212 = event-data() -> ()  [unwired: 3 out]
      }
      event "参数加载": Value Change {
        n213 = event-data() -> ()  [unwired: 7 out]
        n214 = property on="压装轴承，挡圈曲线" class="XYGraph (严格)"("YScale.Maximum"="Y轴承最大值") -> ()  [unwired: 2 in, 2 out]
        n215 = property on="压装轴承，挡圈曲线" class="XYGraph (严格)"("YScale.Minimum"="Y轴承最小值") -> ()  [unwired: 2 in, 2 out]
        n216 = property on="压装轴承，挡圈曲线" class="XYGraph (严格)"("XScale.Maximum"="X轴承最大值") -> ()  [unwired: 2 in, 2 out]
        n217 = property on="压装轴承，挡圈曲线" class="XYGraph (严格)"("XScale.Minimum"="X轴承最小值") -> ()  [unwired: 2 in, 2 out]
        n218 = property on="压装滚针轴承" class="XYGraph (严格)"("XScale.Maximum"="X内圈最大值") -> ()  [unwired: 2 in, 2 out]
        n219 = property on="压装滚针轴承" class="XYGraph (严格)"("XScale.Minimum"="X内圈最小值") -> ()  [unwired: 2 in, 2 out]
        n220 = property on="压装滚针轴承" class="XYGraph (严格)"("YScale.Maximum"="Y内圈最大值") -> ()  [unwired: 2 in, 2 out]
        n221 = property on="压装滚针轴承" class="XYGraph (严格)"("YScale.Minimum"="Y内圈最小值") -> ()  [unwired: 2 in, 2 out]
        n222 = property on="挡圈压铆" class="XYGraph (严格)"("XScale.Minimum"="X挡圈最小值") -> ()  [unwired: 2 in, 2 out]
        n223 = property on="挡圈压铆" class="XYGraph (严格)"("YScale.Minimum"="Y挡圈最小值") -> ()  [unwired: 2 in, 2 out]
        n224 = property on="挡圈压铆" class="XYGraph (严格)"("XScale.Maximum"="X挡圈最大值") -> ()  [unwired: 2 in, 2 out]
        n225 = property on="挡圈压铆" class="XYGraph (严格)"("YScale.Maximum"="Y挡圈最大值") -> ()  [unwired: 2 in, 2 out]
      }
      event "停止": Value Change {
        n226 = event-data() -> ()  [unwired: 7 out]
        n227 = flat-sequence {
          frame #0 {
          }
          frame #1 {
            n228 = Wait Until Next ms Multiple(millisecond multiple=u32 1000 ("毫秒倍数")) -> ()  [unwired: 1 out]
          }
          frame #2 {
            n229 = Quit LabVIEW(quit? (T)=TRUE ("停止？(T)")) -> ()
          }
        }
      }
      event "传感器参数查询": Value Change {
        n230 = event-data() -> ()  [unwired: 7 out]
        n231 = local read "ADODB._Connection Out"() -> (w388:refnum<k7>)
        n232 = call "SQL Execute.vi"("Command Text"="SELECT * FROM 传感器校验表 where ID='1'", "ADODB._Connection In"=w388) -> ("Data"=w389:string[][])  [unwired: 6 in, 3 out]
        n233 = Index Array(array=w389) -> (element=w390:string[])  [unwired: 2 in]
        n234 = Fract/Exp String To Number ("分数/指数字符串至数值转换")(string=w390) -> (number=w391:dbl[])  [unwired: 3 in, 1 out]
        n235 = Index Array(array=w391, index #1=1 ("索引"), index #2=2 ("索引"), index #3=3 ("索引"), index #4=4 ("索引"), index #5=5 ("索引"), index #6=6 ("索引"), index #7=7 ("索引"), index #8=8 ("索引"), index #9=9 ("索引"), index #10=10 ("索引"), index #11=11 ("索引"), index #12=12 ("索引")) -> (element #1=w396:dbl, element #2=w397:dbl, element #3=w398:dbl, element #4=w399:dbl, element #5=w378:dbl, element #6=w377:dbl, element #7=w376:dbl, element #8=w375:dbl, element #9=w374:dbl, element #10=w373:dbl, element #11=w372:dbl, element #12=w371:dbl)
        n236 = local write "轴承压力零点偏移"(w396) -> ()
        n237 = local write "轴承压力比例偏移"(w397) -> ()
        n238 = local write "轴承位移零点偏移"(w398) -> ()
        n239 = local write "轴承位移比例偏移"(w399) -> ()
        n240 = local write "内圈压力零点偏移"(w378) -> ()
        n241 = local write "内圈压力比例偏移"(w377) -> ()
        n242 = local write "内圈位移零点偏移"(w376) -> ()
        n243 = local write "内圈位移比例偏移"(w375) -> ()
        n244 = local write "压铆压力零点偏移"(w374) -> ()
        n245 = local write "压铆压力比例偏移"(w373) -> ()
        n246 = local write "压铆位移零点偏移"(w372) -> ()
        n247 = local write "压铆位移比例偏移"(w371) -> ()
      }
      event "参数查询": Value Change {
        n248 = event-data() -> ()  [unwired: 7 out]
        n249 = flat-sequence {
          tunnel: [w405] -> w400
          tunnel: [w410] -> w402
          tunnel: [w406] -> w401
          tunnel: w400 -> [w408]
          tunnel: w402 -> [w414]
          tunnel: w401 -> [w413]
          frame #0 {
            n250 = local read "ADODB._Connection Out"() -> (w405:refnum<k7>)
            n251 = call-poly <vilib>:"Read From Spreadsheet File.vi"("file path (dialog if empty)"=path "D:/Q14070-B010/参数/参数项.txt") -> ("first row"=w403:string[])  [unwired: 6 in, 4 out]
            n252 = property on="参数浏览表" class="Tbl (严格)"("Row Headers[]"=w403) -> ()  [unwired: 2 in, 2 out]
          }
          frame #1 {
            n253 = call "SQL Execute.vi"("Command Text"="SELECT * FROM 测试参数表;", "ADODB._Connection In"=w408) -> ("error out"=w410:errorcluster, "Data"=w411:string[][])  [unwired: 6 in, 2 out]
            n254 = Transpose 2D Array(2D array=w411) -> (transposed array=w406:string[][])
            n255 = Index Array(array=w406, index (row)=0 ("索引 (行)")) -> (element=w409:string[])  [unwired: 1 in]
            n256 = property on="参数浏览表" class="Tbl (严格)"("Column Headers[]"=w409) -> ()  [unwired: 2 in, 2 out]
          }
          frame #2 {
            n257 = local write "参数浏览表"(w413) -> ()
            "error out 2" <- w414
          }
        }
      }
      event "传感器参数保存": Value Change {
        n258 = event-data() -> ()  [unwired: 7 out]
        n259 = local read "轴承压力零点偏移"() -> (w453:dbl)
        n260 = local read "轴承压力比例偏移"() -> (w452:dbl)
        n261 = local read "轴承位移零点偏移"() -> (w451:dbl)
        n262 = local read "轴承位移比例偏移"() -> (w450:dbl)
        n263 = local read "内圈压力零点偏移"() -> (w449:dbl)
        n264 = local read "内圈压力比例偏移"() -> (w448:dbl)
        n265 = local read "内圈位移零点偏移"() -> (w447:dbl)
        n266 = local read "内圈位移比例偏移"() -> (w446:dbl)
        n267 = local read "压铆压力零点偏移"() -> (w445:dbl)
        n268 = local read "压铆压力比例偏移"() -> (w444:dbl)
        n269 = local read "压铆位移零点偏移"() -> (w443:dbl)
        n270 = local read "压铆位移比例偏移"() -> (w442:dbl)
        n271 = Build Array(w453, w452, w451, w450, w449, w448, w447, w446, w445, w444, w443, w442) -> (w441:dbl[])
        n272 = Number To Fractional String(number=w441, precision (6)=i16 2 ("精度(6)")) -> (F-format string=w439:string[])  [unwired: 2 in]
        n273 = Index Array(array=w439, index #1=0 ("索引"), index #2=1 ("索引"), index #3=2 ("索引"), index #4=3 ("索引"), index #5=4 ("索引"), index #6=5 ("索引"), index #7=6 ("索引"), index #8=7 ("索引"), index #9=8 ("索引"), index #10=9 ("索引"), index #11=10 ("索引"), index #12=11 ("索引")) -> (element #1=w426:string, element #2=w425:string, element #3=w424:string, element #4=w423:string, element #5=w422:string, element #6=w421:string, element #7=w420:string, element #8=w419:string, element #9=w418:string, element #10=w417:string, element #11=w416:string, element #12=w415:string)
        n274 = call "创建文本3"("右压力零点偏移"=w426, "右压力比例偏移"=w425, "右位移零点偏移"=w424, "右位移比例偏移"=w423, "左压力零点偏移"=w422, "左压力比例偏移"=w421, "左位移零点偏移"=w420, "左位移比例偏移"=w419, "压铆压力零点偏移"=w418, "压铆压力比例偏移"=w417, "压铆位移零点偏移"=w416, "压铆位移比例偏移"=w415) -> ("Result"=w455:string)  [unwired: 14 in, 1 out]
        n275 = local read "ADODB._Connection Out"() -> (w454:refnum<k7>)
        n276 = call "SQL Execute.vi"("Command Text"=w455, "ADODB._Connection In"=w454) -> ("error out"=w458:errorcluster, "ADODB._Connection Out"=w457:refnum<k7>)  [unwired: 6 in, 2 out]
        n277 = call "ADO Connection Close.vi"("error in (no error)"=w458, "ADODB._Connection In"=w457) -> ("error out"=→"error out 3":errorcluster)  [unwired: 8 in, 1 out]
      }
      event "试验参数保存": Value Change {
        n278 = event-data() -> ()  [unwired: 7 out]
        n279 = while {
          i -> [w463]
          stop <- w462 stop-if-true
          n280 = local read "型号数量"() -> (w460:i32)
          n281 = Wait Until Next ms Multiple(millisecond multiple=u32 50 ("毫秒倍数")) -> ()  [unwired: 1 out]
          n282 = Greater Or Equal?(x=w463, y=w460) -> (x >= y?=w462:bool)
          n283 = Index Array(array="参数浏览表", index (col)=w463) -> (element=w469:string[])  [unwired: 1 in]
          n284 = stacked-sequence "层叠式顺序结构" {
            seq-local: [w470 _ _ _] -> [_ w502 _ _]
            seq-local: [_ w504 _ _] -> [_ _ w532 _]
            seq-local: [_ _ w533 _] -> [_ _ _ w560]
            tunnel: w469 -> [w501 w505 w546 w592]
            tunnel: [_ _ _ w561] -> w459
            frame #0 {
              n285 = Index Array(array=w501, index #2=2 ("索引"), index #3=3 ("索引"), index #4=4 ("索引"), index #5=5 ("索引"), index #6=6 ("索引"), index #7=7 ("索引"), index #8=8 ("索引"), index #9=9 ("索引"), index #10=10 ("索引"), index #11=11 ("索引"), index #12=12 ("索引"), index #13=13 ("索引"), index #14=14 ("索引"), index #15=15 ("索引"), index #16=16 ("索引")) -> (element #2=w485:string, element #3=w484:string, element #4=w483:string, element #5=w482:string, element #6=w481:string, element #7=w480:string, element #8=w479:string, element #9=w478:string, element #10=w477:string, element #11=w476:string, element #12=w475:string, element #13=w474:string, element #14=w473:string, element #15=w472:string, element #16=w471:string)  [unwired: 1 in, 1 out]
              n286 = call "创建文本5"("1监控点"=w485, "1监控点最小压力"=w484, "1监控点最大压力"=w483, "1最小压装位移"=w482, "1最大压装位移"=w481, "2监控点"=w480, "2监控点最小压力"=w479, "2监控点最大压力"=w478, "2最小压装位移"=w477, "2最大压装位移"=w476, "3监控点"=w475, "3监控点最小压力"=w474, "3监控点最大压力"=w473, "3最小压装位移"=w472, "3最大压装位移"=w471) -> ("Result"=w470:string)  [unwired: 11 in, 1 out]
            }
            frame #1 {
              n287 = Index Array(array=w505, index #2=29 ("索引"), index #3=30 ("索引"), index #4=31 ("索引"), index #5=32 ("索引"), index #6=33 ("索引"), index #7=34 ("索引"), index #8=35 ("索引"), index #9=36 ("索引"), index #10=37 ("索引"), index #11=38 ("索引"), index #12=39 ("索引"), index #13=40 ("索引"), index #14=0 ("索引")) -> (element #2=w517:string, element #3=w516:string, element #4=w515:string, element #5=w514:string, element #6=w513:string, element #7=w512:string, element #8=w511:string, element #9=w510:string, element #10=w509:string, element #11=w508:string, element #12=w507:string, element #13=w506:string)  [unwired: 2 in, 3 out]
              n288 = call "创建文本2"("1区域最小位移"=w517, "1区域最大位移"=w516, "1区域最小压力"=w515, "1区域最大压力"=w514, "2区域最小位移"=w513, "2区域最大位移"=w512, "2区域最小压力"=w511, "2区域最大压力"=w510, "3区域最小位移"=w509, "3区域最大位移"=w508, "3区域最小压力"=w507, "3区域最大压力"=w506) -> ("Result"=w503:string)  [unwired: 14 in, 1 out]
              n289 = Concatenate Strings(w502, w503) -> (w504:string)
            }
            frame #2 {
              n290 = Index Array(array=w546, index #2=43 ("索引"), index #3=44 ("索引"), index #4=45 ("索引"), index #5=46 ("索引"), index #6=47 ("索引"), index #7=48 ("索引"), index #8=49 ("索引"), index #9=50 ("索引"), index #10=51 ("索引"), index #11=52 ("索引"), index #12=53 ("索引"), index #13=54 ("索引")) -> (element #2=w545:string, element #3=w544:string, element #4=w543:string, element #5=w542:string, element #6=w541:string, element #7=w540:string, element #8=w539:string, element #9=w538:string, element #10=w537:string, element #11=w536:string, element #12=w535:string, element #13=w534:string)  [unwired: 3 in, 3 out]
              n291 = call "创建文本6"("X轴承最小值"=w545, "X轴承最大值"=w544, "Y轴承最小值"=w543, "Y轴承最大值"=w542, "X内圈最小值"=w541, "X内圈最大值"=w540, "Y内圈最小值"=w539, "Y内圈最大值"=w538, "X挡圈最小值"=w537, "X挡圈最大值"=w536, "Y挡圈最小值"=w535, "Y挡圈最大值"=w534) -> ("Result"=w531:string)  [unwired: 14 in, 1 out]
              n292 = Concatenate Strings(w532, w531) -> (w533:string)
            }
            frame #3 {
              n293 = Index Array(array=w592, index #1=0 ("索引"), index #2=17 ("索引"), index #3=18 ("索引"), index #4=19 ("索引"), index #5=20 ("索引"), index #6=21 ("索引"), index #7=22 ("索引"), index #8=23 ("索引"), index #9=24 ("索引"), index #10=25 ("索引"), index #11=26 ("索引"), index #12=27 ("索引"), index #13=28 ("索引"), index #14=41 ("索引"), index #15=42 ("索引")) -> (element #1=w564:string, element #2=w578:string, element #3=w577:string, element #4=w576:string, element #5=w575:string, element #6=w574:string, element #7=w573:string, element #8=w572:string, element #9=w571:string, element #10=w570:string, element #11=w569:string, element #12=w568:string, element #13=w567:string, element #14=w563:string, element #15=w562:string)
              n294 = call "创建文本4"("1快下位置"=w578, "1快下速度"=w577, "1慢下位置"=w576, "1慢下速度"=w575, "1快上位置"=w574, "1快上速度"=w573, "2快下位置"=w572, "2快下速度"=w571, "2慢下位置"=w570, "2慢下速度"=w569, "2快上位置"=w568, "2快上速度"=w567, "压轴承换向力"=w563, "压内圈换向力"=w562, "产品型号"=w564) -> ("Result"=w559:string)  [unwired: 11 in, 1 out]
              n295 = Concatenate Strings(w560, w559) -> (w561:string)
            }
          }
          n296 = local read "ADODB._Connection Out"() -> (w461:refnum<k7>)
          n297 = call "SQL Execute.vi"("Command Text"=w459, "ADODB._Connection In"=w461) -> ("error out"=w467:errorcluster, "ADODB._Connection Out"=w468:refnum<k7>)  [unwired: 6 in, 2 out]
          n298 = call "ADO Connection Close.vi"("error in (no error)"=w467, "ADODB._Connection In"=w468) -> ("error out"=→"error out 4":errorcluster)  [unwired: 8 in, 1 out]
        }
      }
    }
    n299 = local read "停止"() -> (w354:bool)
    n300 = Wait Until Next ms Multiple(millisecond multiple=u32 50 ("毫秒倍数")) -> ()  [unwired: 1 out]
  }
  n301 = flat-sequence {
    tunnel: [w596] -> w4
    tunnel: [w594] -> w3
    tunnel: w4 -> [w601]
    tunnel: w3 -> [w600]
    tunnel: [w599] -> w2
    tunnel: [w598] -> w1
    tunnel: w2 -> [w831]
    tunnel: w1 -> [w830]
    frame #0 {
      n302 = call "ADO Connection Create.vi"() -> ("error out"=w595:errorcluster, "ADODB._Connection Out"=w597:refnum<k7>)  [unwired: 10 in]
      n303 = call "ADO Connection Open.vi"("error in (no error)"=w595, "ConnectionString"="Provider=Microsoft.Jet.OLEDB.4.0;Data Source=D:\\Q14070-B010\\参数\\参数B010.mdb;Persist Security Info=False;Jet OLEDB:Database Password=123;", "ADODB._Connection In"=w597) -> ("error out"=w594:errorcluster, "ADODB._Connection Out"=w596:refnum<k7>)  [unwired: 7 in]
    }
    frame #1 {
      n304 = while {
        tunnel: w601 -> [w605]
        tunnel: w600 -> [w604]
        tunnel: [w603] -> w599
        tunnel: [w602] -> w598
        stop <- w606 stop-if-true
        n305 = stacked-sequence {
          tunnel: w605 -> [w611 _ _ _ _]
          tunnel: w604 -> [w610 _ _ _ _]
          tunnel: [w608 _ _ _ _] -> w603
          tunnel: [w609 _ _ _ _] -> w602
          frame #0 {
            n306 = local read "参数加载"() -> (w613:bool)
            n307 = First Call?() -> (First Call?: T/F=w614:bool)
            n308 = Or(x=w614, y=w613) -> (x .or. y?=w612:bool)
            n309 = case shown="真" w612 {
              tunnel: w611 -> [_ w618]
              tunnel: w610 -> [_ w617]
              tunnel: [_ w616] -> w609
              tunnel: [_ w615] -> w608
              frame False {
              }
              frame True {
                n310 = stacked-sequence {
                  seq-local: [w624 _ _] -> [_ w645 _]
                  seq-local: [w623 _ _] -> [_ w643 _]
                  tunnel: w618 -> [w629 _ _]
                  tunnel: w617 -> [w626 _ _]
                  tunnel: [_ w644 _] -> w616
                  tunnel: [_ w642 _] -> w615
                  frame #0 {
                    n311 = call "SQL Execute.vi"("error in (no error)"=w626, "Command Text"="SELECT * FROM 测试参数表 ;  ", "ADODB._Connection In"=w629) -> ("error out"=w624:errorcluster, "Data"=w628:string[][], "ADODB._Connection Out"=w623:refnum<k7>)  [unwired: 5 in, 1 out]
                    n312 = Index Array(array=w628, index (col)=0 ("索引 (行)")) -> (element=w621:string[])  [unwired: 1 in]
                    n313 = Array Size(array=w621) -> (size(s)=w620:i32)
                    "型号数量" <- w620
                    n314 = while {
                      shift-right: [w635] -> w619
                      shift-left: i32[] [] -> [w634]
                      tunnel: w620 -> [w632]
                      i -> [w633]
                      stop <- w631 stop-if-true
                      n315 = Greater Or Equal?(x=w633, y=w632) -> (x >= y?=w631:bool)
                      n316 = Build Array (concatenate)(w634, w633) -> (w635:i32[])
                    }
                    n317 = Build Cluster Array "索引与捆绑簇数组"(w621, w619) -> (w627:cluster{"String":string, i32}[])
                    n318 = property on="型号选择" class="Ring (严格)"("StringsAndValues[]"=w627) -> ()  [unwired: 2 in, 2 out]
                  }
                  frame #1 {
                    n319 = property on="型号选择" class="Ring (严格)"() -> ("RingText.Text"=w640:string)  [unwired: 2 in, 2 out]
                    n320 = call "创建文本"("型号选择"=w640) -> ("Result"=w641:string)  [unwired: 13 in, 1 out]
                    n321 = call "SQL Execute.vi"("error in (no error)"=w645, "Command Text"=w641, "ADODB._Connection In"=w643) -> ("error out"=w644:errorcluster, "Data"=w639:string[][], "ADODB._Connection Out"=w642:refnum<k7>)  [unwired: 5 in, 1 out]
                    n322 = Index Array(array=w639, index (row)=0 ("索引 (行)")) -> (element=w637:string[])  [unwired: 1 in]
                    n323 = Fract/Exp String To Number ("分数/指数字符串至数值转换")(string=w637) -> (number=w636:dbl[])  [unwired: 3 in, 1 out]
                    n324 = stacked-sequence {
                      tunnel: w636 -> [w676 w701 w726 w755]
                      frame #0 {
                        n325 = Index Array ("索引数组")(array=w676, index #1=2 ("索引"), index #2=3 ("索引"), index #3=4 ("索引"), index #4=5 ("索引"), index #5=6 ("索引"), index #6=7 ("索引"), index #7=8 ("索引"), index #8=9 ("索引"), index #9=10 ("索引"), index #10=11 ("索引"), index #11=12 ("索引"), index #12=13 ("索引"), index #13=14 ("索引"), index #14=15 ("索引"), index #15=16 ("索引")) -> (element #1=w675:dbl, element #2=w674:dbl, element #3=w673:dbl, element #4=w672:dbl, element #5=w671:dbl, element #6=w670:dbl, element #7=w669:dbl, element #8=w668:dbl, element #9=w667:dbl, element #10=w666:dbl, element #11=w665:dbl, element #12=w664:dbl, element #13=w663:dbl, element #14=w662:dbl, element #15=w661:dbl)
                        n326 = local write "内圈最小压装位移(mm)"(w667) -> ()
                        n327 = local write "轴承最大压装位移(mm)"(w671) -> ()
                        n328 = local write "轴承最小压装位移(mm)"(w672) -> ()
                        n329 = local write "内圈最大压装位移(mm)"(w666) -> ()
                        n330 = local write "轴承监控点"(w675) -> ()
                        n331 = local write "内圈最大压力(N)"(w668) -> ()
                        n332 = local write "内圈监控点"(w670) -> ()
                        n333 = local write "轴承最小压力(N)"(w674) -> ()
                        n334 = local write "内圈最小压力(N)"(w669) -> ()
                        n335 = local write "轴承最大压力(N)"(w673) -> ()
                        n336 = local write "3最小压装位移"(w662) -> ()
                        n337 = local write "压铆最大压力(N)"(w663) -> ()
                        n338 = local write "压铆最小压力(N)"(w664) -> ()
                        n339 = local write "3最大压装位移"(w661) -> ()
                        n340 = local write "3监控点"(w665) -> ()
                      }
                      frame #1 {
                        n341 = Index Array(array=w701, index #1=17 ("索引"), index #2=18 ("索引"), index #3=19 ("索引"), index #4=20 ("索引"), index #5=21 ("索引"), index #6=22 ("索引"), index #7=23 ("索引"), index #8=24 ("索引"), index #9=25 ("索引"), index #10=26 ("索引"), index #11=27 ("索引"), index #12=28 ("索引")) -> (element #1=w688:dbl, element #2=w687:dbl, element #3=w686:dbl, element #4=w685:dbl, element #5=w684:dbl, element #6=w683:dbl, element #7=w682:dbl, element #8=w681:dbl, element #9=w680:dbl, element #10=w679:dbl, element #11=w678:dbl, element #12=w677:dbl)
                        n342 = local write "慢速下降速度"(w685) -> ()
                        n343 = local write "快速上升位置"(w684) -> ()
                        n344 = local write "快速下降速度"(w687) -> ()
                        n345 = local write "慢速下降位置"(w686) -> ()
                        n346 = local write "快速上升速度"(w683) -> ()
                        n347 = local write "快速下降位置"(w688) -> ()
                        n348 = local write "快速下降位置"(w682) -> ()
                        n349 = local write "慢速下降速度"(w679) -> ()
                        n350 = local write "快速上升位置"(w678) -> ()
                        n351 = local write "快速下降速度"(w681) -> ()
                        n352 = local write "慢速下降位置"(w680) -> ()
                        n353 = local write "快速上升速度"(w677) -> ()
                      }
                      frame #2 {
                        n354 = Index Array(array=w726, index #1=29 ("索引"), index #2=30 ("索引"), index #3=31 ("索引"), index #4=32 ("索引"), index #5=33 ("索引"), index #6=34 ("索引"), index #7=35 ("索引"), index #8=36 ("索引"), index #9=37 ("索引"), index #10=38 ("索引"), index #11=39 ("索引"), index #12=40 ("索引")) -> (element #1=w713:dbl, element #2=w712:dbl, element #3=w711:dbl, element #4=w710:dbl, element #5=w709:dbl, element #6=w708:dbl, element #7=w707:dbl, element #8=w706:dbl, element #9=w705:dbl, element #10=w704:dbl, element #11=w703:dbl, element #12=w702:dbl)
                        n355 = local write "挡圈区域最小压力(N)"(w703) -> ()
                        n356 = local write "挡圈区域最大压力(N)"(w702) -> ()
                        n357 = local write "挡圈区域最小位移(mm)"(w705) -> ()
                        n358 = local write "挡圈区域最大位移(mm)"(w704) -> ()
                        n359 = local write "轴承区域最小位移(mm)"(w713) -> ()
                        n360 = local write "轴承区域最大位移(mm)"(w712) -> ()
                        n361 = local write "内圈区域最小压力(N)"(w707) -> ()
                        n362 = local write "内圈区域最大压力(N)"(w706) -> ()
                        n363 = local write "轴承区域最小压力(N)"(w711) -> ()
                        n364 = local write "轴承区域最大压力(N)"(w710) -> ()
                        n365 = local write "内圈区域最小位移(mm)"(w709) -> ()
                        n366 = local write "内圈区域最大位移(mm)"(w708) -> ()
                      }
                      frame #3 {
                        n367 = Index Array(array=w755, index #1=41 ("索引"), index #2=42 ("索引"), index #3=43 ("索引"), index #4=44 ("索引"), index #5=45 ("索引"), index #6=46 ("索引"), index #7=47 ("索引"), index #8=48 ("索引"), index #9=49 ("索引"), index #10=50 ("索引"), index #11=51 ("索引"), index #12=52 ("索引"), index #13=53 ("索引"), index #14=54 ("索引")) -> (element #1=w751:dbl, element #2=w752:dbl, element #3=w738:dbl, element #4=w737:dbl, element #5=w736:dbl, element #6=w735:dbl, element #7=w734:dbl, element #8=w733:dbl, element #9=w732:dbl, element #10=w731:dbl, element #11=w730:dbl, element #12=w729:dbl, element #13=w728:dbl, element #14=w727:dbl)
                        n368 = local write "压轴承换向压力"(w751) -> ()
                        n369 = local write "换向压力2"(w752) -> ()
                        n370 = local write "X内圈最小值"(w734) -> ()
                        n371 = local write "X内圈最大值"(w733) -> ()
                        n372 = local write "Y内圈最小值"(w732) -> ()
                        n373 = local write "Y内圈最大值"(w731) -> ()
                        n374 = local write "X轴承最小值"(w738) -> ()
                        n375 = local write "X轴承最大值"(w737) -> ()
                        n376 = local write "Y轴承最小值"(w736) -> ()
                        n377 = local write "Y轴承最大值"(w735) -> ()
                        n378 = local write "X挡圈最小值"(w730) -> ()
                        n379 = local write "X挡圈最大值"(w729) -> ()
                        n380 = local write "Y挡圈最小值"(w728) -> ()
                        n381 = local write "Y挡圈最大值"(w727) -> ()
                      }
                    }
                  }
                  frame #2 {
                    n382 = local read "ADODB._Connection Out"() -> (w773:refnum<k7>)
                    n383 = call "SQL Execute.vi"("Command Text"="SELECT * FROM 传感器校验表 where ID='1'", "ADODB._Connection In"=w773) -> ("Data"=w774:string[][])  [unwired: 6 in, 3 out]
                    n384 = Index Array(array=w774) -> (element=w775:string[])  [unwired: 2 in]
                    n385 = Fract/Exp String To Number ("分数/指数字符串至数值转换")(string=w775) -> (number=w776:dbl[])  [unwired: 3 in, 1 out]
                    n386 = Index Array(array=w776, index #1=1 ("索引"), index #2=2 ("索引"), index #3=3 ("索引"), index #4=4 ("索引"), index #5=5 ("索引"), index #6=6 ("索引"), index #7=7 ("索引"), index #8=8 ("索引"), index #9=9 ("索引"), index #10=10 ("索引"), index #11=11 ("索引"), index #12=12 ("索引")) -> (element #1=w781:dbl, element #2=w782:dbl, element #3=w783:dbl, element #4=w784:dbl, element #5=w763:dbl, element #6=w762:dbl, element #7=w761:dbl, element #8=w760:dbl, element #9=w759:dbl, element #10=w758:dbl, element #11=w757:dbl, element #12=w756:dbl)
                    n387 = local write "轴承压力零点偏移"(w781) -> ()
                    n388 = local write "轴承压力比例偏移"(w782) -> ()
                    n389 = local write "轴承位移零点偏移"(w783) -> ()
                    n390 = local write "轴承位移比例偏移"(w784) -> ()
                    n391 = local write "内圈压力零点偏移"(w763) -> ()
                    n392 = local write "内圈压力比例偏移"(w762) -> ()
                    n393 = local write "内圈位移零点偏移"(w761) -> ()
                    n394 = local write "内圈位移比例偏移"(w760) -> ()
                    n395 = local write "压铆压力零点偏移"(w759) -> ()
                    n396 = local write "压铆压力比例偏移"(w758) -> ()
                    n397 = local write "压铆位移零点偏移"(w757) -> ()
                    n398 = local write "压铆位移比例偏移"(w756) -> ()
                  }
                }
              }
            }
            "ADODB._Connection Out" <- w611
          }
          frame #1 {
            n399 = First Call?() -> (First Call?: T/F=w785:bool)
            n400 = case shown="真" w785 {
              frame False {
              }
              frame True {
                n401 = call "员工管理测试程序.vi"() -> ("员工姓名"=w787:string, "员工ID"=w786:string)  [unwired: 10 in]
                n402 = local write "员工ID"(w786) -> ()
                n403 = local write "员工姓名"(w787) -> ()
              }
            }
          }
          frame #2 {
          }
          frame #3 {
            n404 = local read "报警工步号"() -> (w789:dbl)
            n405 = local read "自动工步号"() -> (w791:dbl)
            n406 = case shown="1" w789 {
              tunnel: ["轴承不在位" ("工步操作状态") "触碰光幕，请复位" ("工步操作状态") _ "压装1不合格" ("工步操作状态")] -> w788
              frame 1 {
              }
              frame 2 {
              }
              frame 0, Default {
              }
              frame 6 {
              }
            }
            "报警提示" <- w788
            n407 = case shown="5" w791 {
              tunnel: [w795 "轴承不在位，或者装反，按复位解除报警" ("工步操作状态") "压装1不合格" ("工步操作状态") "压装2不合格" ("工步操作状态") "压装3不合格" ("工步操作状态") "请释放急停按钮" ("工步操作状态") "伺服1快下" ("工步操作状态") "伺服1慢下" ("工步操作状态") "保压中" ("工步操作状态") "伺服1快速上升" ("工步操作状态") "滑台左移" ("工步操作状态") "伺服2快下" ("工步操作状态") "伺服2慢下" ("工步操作状态") "伺服2慢下" ("工步操作状态") "保压中" ("工步操作状态") "伺服2快速上升" ("工步操作状态") "压铆启动" ("工步操作状态") "等待开始增压" ("工步操作状态") "保压" ("工步操作状态") "泄压" ("工步操作状态") "压铆上升，右移" ("工步操作状态") "请取挡圈" ("工步操作状态") "涂脂" ("工步操作状态") "压装不合格" ("工步操作状态") "数据上传完成" ("工步操作状态")] -> w790
              frame 0, Default {
                n408 = local read "联线按钮"() -> (w796:bool)
                n409 = case shown="真" w796 {
                  tunnel: ["等待工件" ("工步操作状态") "等待扫描条码" ("工步操作状态")] -> w795
                  frame False {
                  }
                  frame True {
                  }
                }
              }
              frame 5 {
              }
              frame 6 {
              }
              frame 7 {
              }
              frame 8 {
              }
              frame 9 {
              }
              frame 10 {
              }
              frame 20 {
              }
              frame 30 {
              }
              frame 40 {
              }
              frame 50 {
              }
              frame 60 {
              }
              frame 65 {
              }
              frame 70 {
              }
              frame 80 {
              }
              frame 90 {
              }
              frame 100 {
              }
              frame 120 {
              }
              frame 130 {
              }
              frame 140 {
              }
              frame 150 {
              }
              frame 170 {
              }
              frame 180 {
              }
              frame 800 {
              }
              frame 900 {
              }
            }
            "自动操作状态" <- w790
          }
          frame #4 {
            n410 = flat-sequence {
              frame #0 {
                n411 = First Call?() -> (First Call?: T/F=w823:bool)
                n412 = case shown="真" w823 {
                  frame False {
                  }
                  frame True {
                    n413 = local write "B010本序不合格"(FALSE ("B010本序不合格")) -> ()
                    n414 = local write "B010本序合格"(TRUE ("B010本序合格")) -> ()
                  }
                }
              }
              frame #1 {
                n415 = while {
                  stop <- w827 stop-if-true
                  n416 = local read "B010本序不合格"() -> (w826:bool)
                  n417 = case shown="真" w826 {
                    frame False {
                    }
                    frame True {
                      n418 = call "显示对话框信息"() -> ()  [unwired: 10 in, 2 out]
                    }
                  }
                  n419 = local read "B010本序合格"() -> (w827:bool)
                  n420 = Wait Until Next ms Multiple(millisecond multiple=u32 50 ("毫秒倍数")) -> ()  [unwired: 1 out]
                }
              }
            }
          }
        }
        n421 = Wait Until Next ms Multiple(millisecond multiple=u32 50 ("毫秒倍数")) -> ()  [unwired: 1 out]
        n422 = local read "停止"() -> (w606:bool)
      }
    }
    frame #2 {
      n423 = call "ADO Connection Close.vi"("error in (no error)"=w830, "ADODB._Connection In"=w831) -> ("error out"=→"error out":errorcluster)  [unwired: 8 in, 1 out]
    }
  }
  n424 = flat-sequence {
    tunnel: [w832] -> w7
    tunnel: w7 -> [w834]
    tunnel: [w833] -> w6
    tunnel: w6 -> [w922]
    tunnel: [w922] -> w5
    tunnel: w5 -> [w924]
    frame #0 {
      n425 = call "PCI8622配置.vi"() -> ("DeviceID"=w832:i32)  [unwired: 11 in]
    }
    frame #1 {
      n426 = while {
        tunnel: w834 -> [w909]
        tunnel: [w909] -> w833
        stop <- "停止" stop-if-true
        w919 = 0  # nRetSizeWords
        w920 = 2048  # nReadSizeWords
        # "hDevice"
        n427 = Wait Until Next ms Multiple(millisecond multiple=u32 50 ("毫秒倍数")) -> ()  [unwired: 1 out]
        n428 = Initialize Array(u16 0, 2048 ("dimension size")) -> (w910:u16[])
        n429 = dll-call lib="PCI8622_32.dll" fn="PCI8622_ReadDeviceProAD_Npt" label="ReadDeviceProAD_Npt"("hDevice"=w909, "ADBuffer[]"=w910, "nReadSizeWords"=w920, "nRetSizeWords"=w919) -> ("ADBuffer[]"=w913:u16[])  [unwired: 7 in, 2 out]
        n430 = Divide(x=w913, y=65536.01) -> (x/y=w914:dbl[])
        n431 = Multiply(x=w914, y=20) -> (x*y=w917:dbl[])
        n432 = Subtract(x=w917, y=10) -> (x-y=w898:dbl[])
        n433 = Decimate 1D Array "抽取一维数组"(w898) -> (w900:dbl[], w899:dbl[], w906:dbl[], w895:dbl[], w883:dbl[], w882:dbl[])  [unwired: 2 out]
        n434 = Add Array Elements(numeric array=w900) -> (sum=w901:dbl)
        n435 = Add Array Elements(numeric array=w899) -> (sum=w903:dbl)
        n436 = Add Array Elements(numeric array=w906) -> (sum=w907:dbl)
        n437 = Add Array Elements(numeric array=w895) -> (sum=w897:dbl)
        n438 = Array Size(array=w900) -> (size(s)=w902:i32)
        n439 = Array Size(array=w899) -> (size(s)=w904:i32)
        n440 = Array Size(array=w906) -> (size(s)=w905:i32)
        n441 = Array Size(array=w895) -> (size(s)=w896:i32)
        n442 = Add Array Elements(numeric array=w883) -> (sum=w888:dbl)
        n443 = Add Array Elements(numeric array=w882) -> (sum=w886:dbl)
        n444 = Array Size(array=w883) -> (size(s)=w887:i32)
        n445 = Array Size(array=w882) -> (size(s)=w885:i32)
        n446 = Divide(x=w901, y=w902) -> (x/y=w874:dbl)
        n447 = Divide(x=w903, y=w904) -> (x/y=w854:dbl)
        n448 = Divide(x=w907, y=w905) -> (x/y=w856:dbl)
        n449 = Divide(x=w897, y=w896) -> (x/y=w852:dbl)
        n450 = Divide(x=w888, y=w887) -> (x/y=w850:dbl)
        n451 = Divide(x=w886, y=w885) -> (x/y=w847:dbl)
        n452 = local read "内圈压力零点偏移"() -> (w842:dbl)
        n453 = Multiply(x=w847, y=30.0) -> (x*y=w846:dbl)
        n454 = Multiply(x=w852, y=30.0) -> (x*y=w863:dbl)
        n455 = Multiply(x=w856, y=-10000.0) -> (x*y=w866:dbl)
        n456 = local read "压铆压力零点偏移"() -> (w840:dbl)
        n457 = Multiply(x=w874, y=2000.0) -> (x*y=w872:dbl)
        n458 = local read "轴承压力零点偏移"() -> (w890:dbl)
        n459 = local read "压铆位移零点偏移"() -> (w838:dbl)
        n460 = local read "内圈位移零点偏移"() -> (w844:dbl)
        n461 = Multiply(x=w850, y=30.0) -> (x*y=w849:dbl)
        n462 = Multiply(x=w854, y=500.0) -> (x*y=w869:dbl)
        n463 = Subtract(x=w846, y=0.0) -> (x-y=w845:dbl)
        n464 = local read "轴承位移零点偏移"() -> (w836:dbl)
        n465 = Subtract(x=w863, y=0.0) -> (x-y=w851:dbl)
        n466 = Subtract(x=w866, y=90.6) -> (x-y=w855:dbl)
        n467 = Subtract(x=w872, y=515.3) -> (x-y=w857:dbl)
        n468 = local read "压铆压力比例偏移"() -> (w839:dbl)
        n469 = Subtract(x=w849, y=0.0) -> (x-y=w848:dbl)
        n470 = local read "轴承压力比例偏移"() -> (w889:dbl)
        n471 = local read "内圈位移比例偏移"() -> (w843:dbl)
        n472 = local read "轴承位移比例偏移"() -> (w835:dbl)
        n473 = Subtract(x=w869, y=256.8) -> (x-y=w853:dbl)
        n474 = local read "压铆位移比例偏移"() -> (w837:dbl)
        n475 = local read "内圈压力比例偏移"() -> (w841:dbl)
        n476 = Subtract(x=w855, y=w840) -> (x-y=w884:dbl)
        n477 = Subtract(x=w853, y=w842) -> (x-y=w892:dbl)
        n478 = Subtract(x=w848, y=w844) -> (x-y=w880:dbl)
        n479 = Subtract(x=w851, y=w838) -> (x-y=w881:dbl)
        n480 = Subtract(x=w857, y=w890) -> (x-y=w894:dbl)
        n481 = Subtract(x=w845, y=w836) -> (x-y=w879:dbl)
        n482 = Multiply(x=w884, y=w839) -> (x*y=→"压铆压力(N)":dbl)
        n483 = Multiply(x=w894, y=w889) -> (x*y=→"轴承压头压力(N)":dbl)
        n484 = Multiply(x=w892, y=w841) -> (x*y=→"内圈压力(N)":dbl)
        n485 = Multiply(x=w881, y=w837) -> (x*y=→"压铆位移(mm)":dbl)
        n486 = Multiply(x=w880, y=w843) -> (x*y=→"内圈位移(mm)":dbl)
        n487 = Multiply(x=w879, y=w835) -> (x*y=→"轴承压头位移(mm)":dbl)
      }
    }
    frame #2 {
      n488 = dll-call lib="PCI8622_32.dll" fn="PCI8622_StopDeviceProAD" label="StopDeviceProAD"("hDevice"=w922) -> ("hDevice"=w923:i32)  [unwired: 4 in, 2 out]
      n489 = dll-call lib="PCI8622_32.dll" fn="PCI8622_ReleaseDeviceProAD" label="ReleaseDeviceProAD"("hDevice"=w923) -> ()  [unwired: 5 in, 2 out]
    }
    frame #3 {
      n490 = dll-call lib="PCI8622_32.dll" fn="PCI8622_ReleaseDevice" label="ReleaseDevice"("hDevice"=w924) -> ()  [unwired: 5 in, 2 out]
    }
  }
